vi "WriteValue_String.vi"(9 "value":string, 11 "reference":refnum<vi>) -> ()   [LabVIEW 2012]
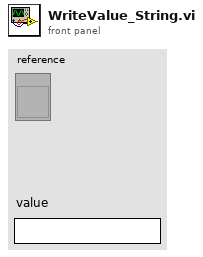
[diagram p1: front panel]
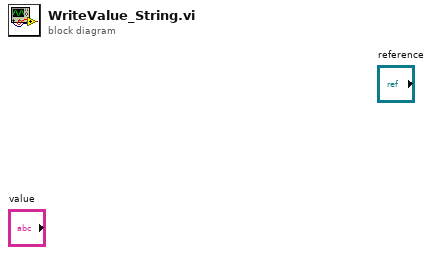
[diagram p0: block diagram]
diagram:
